vi "Time series window-Initialise globals.vi"   [LabVIEW 2020]
uses:
  Globals/gl_Time series viewer globals.vi
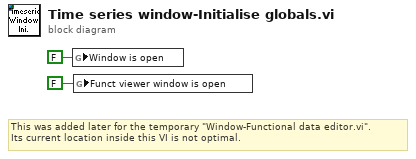
[diagram p0: block diagram]
diagram:
  # "This was added later for the temporary \"Window-Functional data editor.vi\".\nIts current location inside this VI is not optimal."
  n1 = global write "gl_Time series viewer globals.vi" "Window is open"(FALSE ("Bring to front")) -> ()
  n2 = global write "gl_Time series viewer globals.vi" "Funct viewer window is open"(FALSE ("Bring to front")) -> ()
